vi "Check for Fault.vi"(8 "error in (no error)":errorcluster, 11 "SimELoad in":refnum<class "SimEload.lvclass">) -> (0 "error out":errorcluster, 1 "Fault List":string, 2 "Fault Detected?":bool, 3 "SimELoad out":refnum<class "SimEload.lvclass">)   [LabVIEW 2019, in "SimELoad.lvlib" / "SimEload.lvclass"]
uses:
  SimEload.lvclass
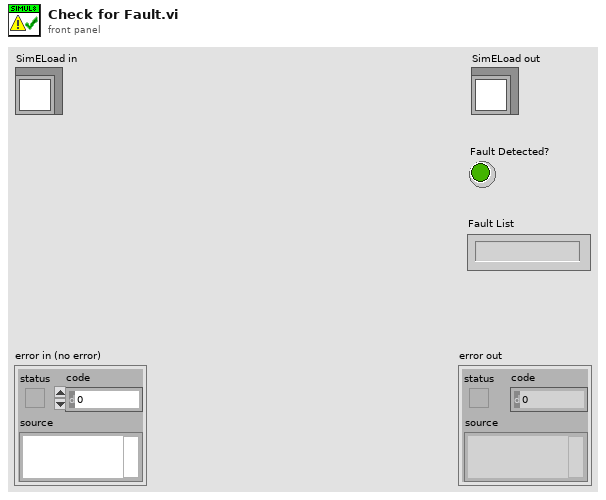
[diagram p1: front panel]
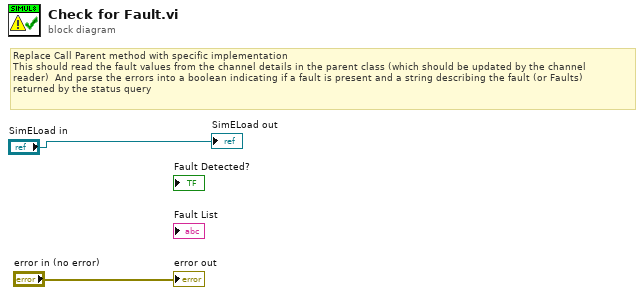
[diagram p0: block diagram]
diagram:
  # "Replace Call Parent method with specific implementation\nThis should read the fault values from the channel details in the parent class (which should be updated by the channel\nreader)  And parse the errors into a boolean indicating if a fault is present and a string describing the fault (or Faults) \nreturned by the status query"
  "error out" <- "error in (no error)"
  "SimELoad out" <- "SimELoad in"
